vi "SQL_OUT Stack Select Cmd.vi"(11 "parameter buffer":T1) -> (3 "连接的字符串":string)   [LabVIEW 2015]
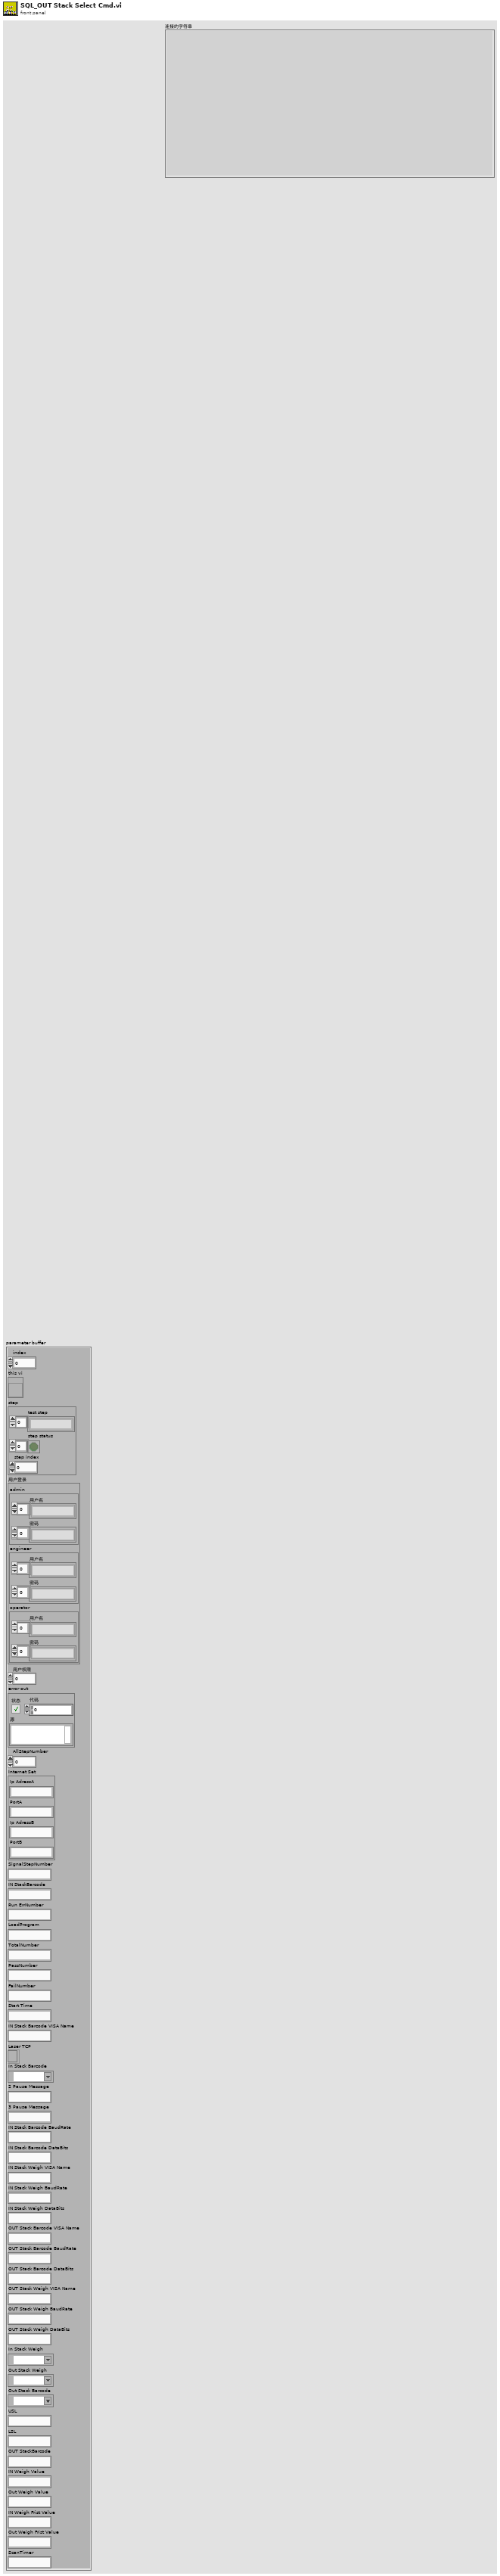
[diagram p1: front panel]
types:
  T1 = cluster{"index":i32, "this vi":refnum<vi>, "step":cluster{"test step":string[], "step status":bool[], "step index":i32}, "用户登录":cluster{"admin":cluster{"用户名":string[], "密码":string[]}, "engineer":cluster{"用户名":string[], "密码":string[]}, "operator":cluster{"用户名":string[], "密码":string[]}}, "用户权限":i32, "error out":errorcluster, "AllStepNumber":i32, "Internet Set":cluster{"Ip AdressA":string, "PortA":string, "Ip AdressB":string, "PortB":string}, "SignalStepNumber":string, "IN StackBarcode":string, "Run ErrNumber":string, "LoadProgram":string, "TotalNumber":string, "PassNumber":string, "FailNumber":string, "Start Time":string, "IN Stack Barcode VISA Name":string, "Laser TCP":refnum<k5>, "In Stack Barcode":refnum<visa-resource-name>, "2 Pause Message":string, "3 Pause Message":string, "IN Stack Barcode BaudRate":string, "IN Stack Barcode DataBits":string, "IN Stack Weigh VISA Name":string, "IN Stack Weigh BaudRate":string, "IN Stack Weigh DataBits":string, "OUT Stack Barcode VISA Name":string, "OUT Stack Barcode BaudRate":string, "OUT Stack Barcode DataBits":string, "OUT Stack Weigh VISA Name":string, "OUT Stack Weigh BaudRate":string, "OUT Stack Weigh DataBits":string, "In Stack Weigh":refnum<visa-resource-name>, "Out Stack Weigh":refnum<visa-resource-name>, "Out Stack Barcode":refnum<visa-resource-name>, "USL":string, "LSL":string, "OUT StackBarcode":string, "IN Weigh Value":string, "Out Weigh Value":string, "IN Weigh Frist Value":string, "Out Weigh Frist Value":string, "ScanTimer":string}
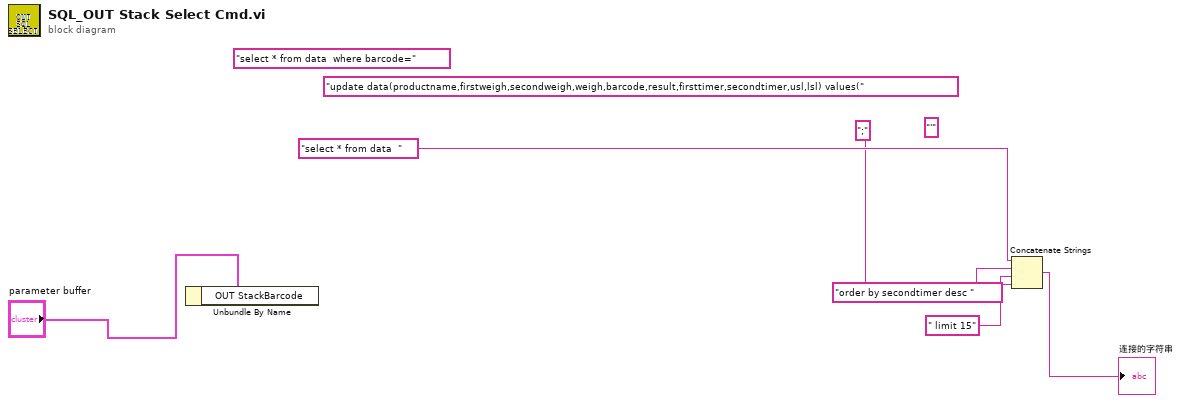
[diagram p0: block diagram]
diagram:
  (unwired) "select * from data  where barcode=" ("字符串")
  (unwired) "update data(productname,firstweigh,secondweigh,weigh,barcode,result,firsttimer,secondtimer,usl,lsl) values(" ("字符串")
  (unwired) "'"
  n1 = Unbundle By Name("parameter buffer") -> ()  [unwired: 1 out]
  n2 = Concatenate Strings("select * from data  " ("字符串"), "order by secondtimer desc " ("字符串"), " limit 15" ("字符串"), ";") -> (→"连接的字符串":string)
